vi "ZCAN_Transmit.vi"(0 "can_index_handle":u32, 1 "协议":u32(ring) items=["CAN", "CANFD"], 3 "ZCAN_Transmit_Data":T2, 5 "error in (no error)":errorcluster caption="错误输入（无错误）", 9 "ZCAN_TransmitFD_Data":T1) -> (19 "error out":errorcluster caption="错误输出")   [LabVIEW 2018]
doc: "该函数用于发送CAN报文。"
uses:
  data_type/ZCAN_Transmit_Data.ctl
  data_type/ZCAN_TransmitFD_Data.ctl
panel:
  in  "每次发送帧数（默认1）":u32=1
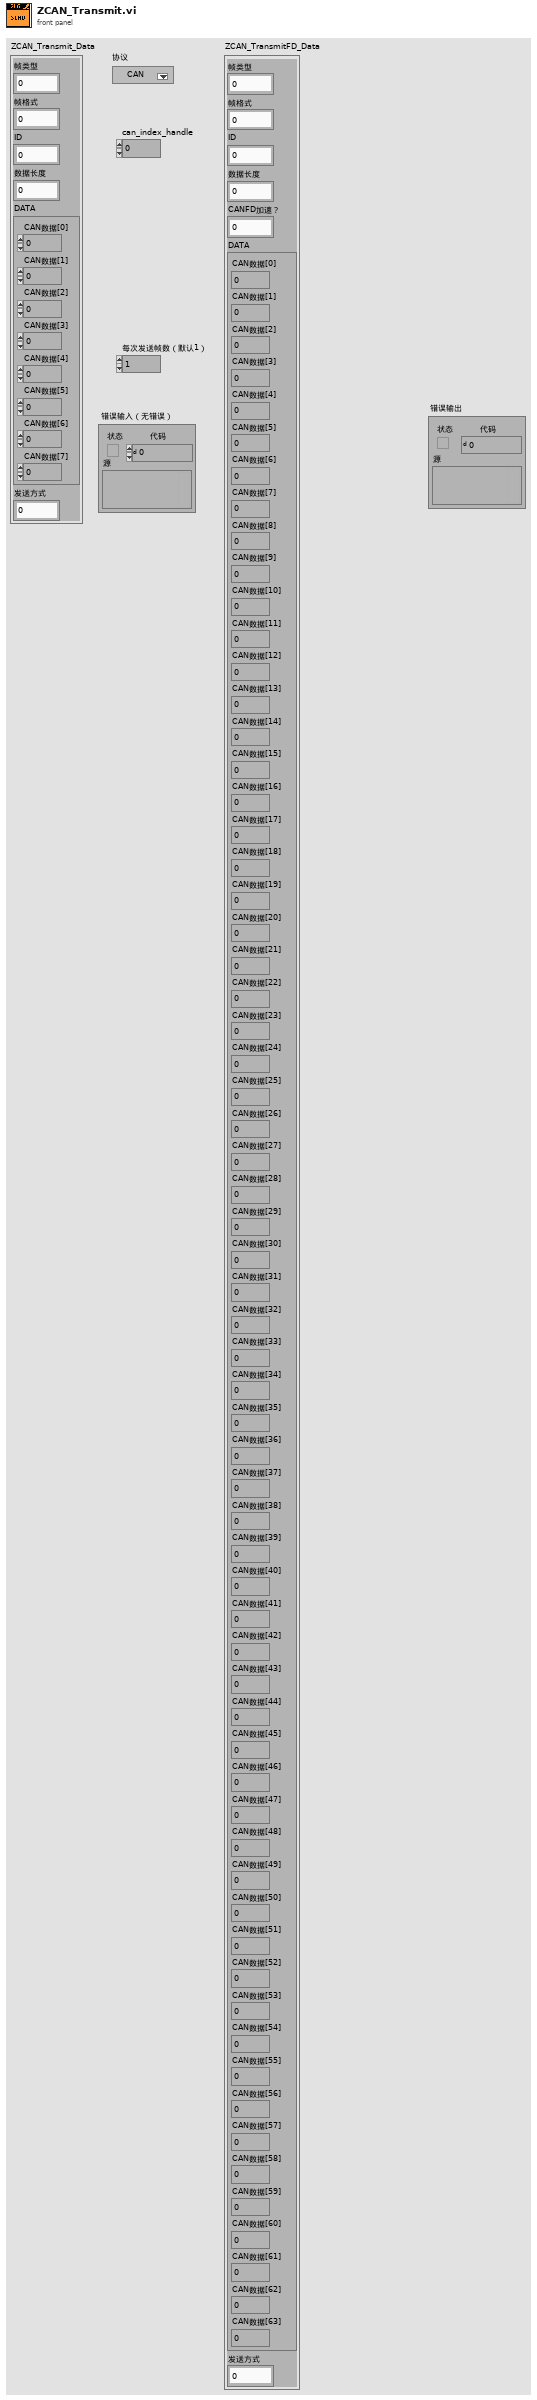
[diagram p1: front panel]
types:
  T1 = typedef "ZCAN_TransmitFD_Data.ctl" = cluster{"帧类型":u32, "帧格式":u32, "ID":u32, "数据长度":u8, "CANFD加速？":u8, "DATA":cluster{"CAN数据[0]":u8, "CAN数据[1]":u8, "CAN数据[2]":u8, "CAN数据[3]":u8, "CAN数据[4]":u8, "CAN数据[5]":u8, "CAN数据[6]":u8, "CAN数据[7]":u8, "CAN数据[8]":u8, "CAN数据[9]":u8, "CAN数据[10]":u8, "CAN数据[11] ":u8, "CAN数据[12] ":u8, "CAN数据[13] ":u8, "CAN数据[14] ":u8, "CAN数据[15] ":u8, "CAN数据[16]":u8, "CAN数据[17]":u8, "CAN数据[18]":u8, "CAN数据[19]":u8, "CAN数据[20]":u8, "CAN数据[21]":u8, "CAN数据[22]":u8, "CAN数据[23]":u8, "CAN数据[24] ":u8, "CAN数据[25]":u8, "CAN数据[26]":u8, "CAN数据[27]":u8, "CAN数据[28]":u8, "CAN数据[29]":u8, "CAN数据[30]":u8, "CAN数据[31]":u8, "CAN数据[32]":u8, "CAN数据[33]":u8, "CAN数据[34]":u8, "CAN数据[35]":u8, "CAN数据[36]":u8, "CAN数据[37]":u8, "CAN数据[38]":u8, "CAN数据[39]":u8, "CAN数据[40]":u8, "CAN数据[41]":u8, "CAN数据[42]":u8, "CAN数据[43]":u8, "CAN数据[44]":u8, "CAN数据[45]":u8, "CAN数据[46]":u8, "CAN数据[47]":u8, "CAN数据[48]":u8, "CAN数据[49]":u8, "CAN数据[50]":u8, "CAN数据[51]":u8, "CAN数据[52]":u8, "CAN数据[53]":u8, "CAN数据[54]":u8, "CAN数据[55]":u8, "CAN数据[56]":u8, "CAN数据[57]":u8, "CAN数据[58]":u8, "CAN数据[59]":u8, "CAN数据[60]":u8, "CAN数据[61]":u8, "CAN数据[62]":u8, "CAN数据[63]":u8}, "发送方式":u32}
  T2 = typedef "ZCAN_Transmit_Data.ctl" = cluster{"帧类型":u32, "帧格式":u32, "ID":u32, "数据长度":u8, "DATA":cluster{"CAN数据[0]":u8, "CAN数据[1]":u8, "CAN数据[2]":u8, "CAN数据[3]":u8, "CAN数据[4]":u8, "CAN数据[5]":u8, "CAN数据[6]":u8, "CAN数据[7]":u8}, "发送方式":u32}
  T3 = cluster{"CAN数据[0]":u8, "CAN数据[1]":u8, "CAN数据[2]":u8, "CAN数据[3]":u8, "CAN数据[4]":u8, "CAN数据[5]":u8, "CAN数据[6]":u8, "CAN数据[7]":u8, "CAN数据[8]":u8, "CAN数据[9]":u8, "CAN数据[10]":u8, "CAN数据[11] ":u8, "CAN数据[12] ":u8, "CAN数据[13] ":u8, "CAN数据[14] ":u8, "CAN数据[15] ":u8, "CAN数据[16]":u8, "CAN数据[17]":u8, "CAN数据[18]":u8, "CAN数据[19]":u8, "CAN数据[20]":u8, "CAN数据[21]":u8, "CAN数据[22]":u8, "CAN数据[23]":u8, "CAN数据[24] ":u8, "CAN数据[25]":u8, "CAN数据[26]":u8, "CAN数据[27]":u8, "CAN数据[28]":u8, "CAN数据[29]":u8, "CAN数据[30]":u8, "CAN数据[31]":u8, "CAN数据[32]":u8, "CAN数据[33]":u8, "CAN数据[34]":u8, "CAN数据[35]":u8, "CAN数据[36]":u8, "CAN数据[37]":u8, "CAN数据[38]":u8, "CAN数据[39]":u8, "CAN数据[40]":u8, "CAN数据[41]":u8, "CAN数据[42]":u8, "CAN数据[43]":u8, "CAN数据[44]":u8, "CAN数据[45]":u8, "CAN数据[46]":u8, "CAN数据[47]":u8, "CAN数据[48]":u8, "CAN数据[49]":u8, "CAN数据[50]":u8, "CAN数据[51]":u8, "CAN数据[52]":u8, "CAN数据[53]":u8, "CAN数据[54]":u8, "CAN数据[55]":u8, "CAN数据[56]":u8, "CAN数据[57]":u8, "CAN数据[58]":u8, "CAN数据[59]":u8, "CAN数据[60]":u8, "CAN数据[61]":u8, "CAN数据[62]":u8, "CAN数据[63]":u8}
  T4 = cluster{u32, "数据长度":u8, "CANFD加速？":u8, u8, u8, "DATA":cluster{"CAN数据[0]":u8, "CAN数据[1]":u8, "CAN数据[2]":u8, "CAN数据[3]":u8, "CAN数据[4]":u8, "CAN数据[5]":u8, "CAN数据[6]":u8, "CAN数据[7]":u8, "CAN数据[8]":u8, "CAN数据[9]":u8, "CAN数据[10]":u8, "CAN数据[11] ":u8, "CAN数据[12] ":u8, "CAN数据[13] ":u8, "CAN数据[14] ":u8, "CAN数据[15] ":u8, "CAN数据[16]":u8, "CAN数据[17]":u8, "CAN数据[18]":u8, "CAN数据[19]":u8, "CAN数据[20]":u8, "CAN数据[21]":u8, "CAN数据[22]":u8, "CAN数据[23]":u8, "CAN数据[24] ":u8, "CAN数据[25]":u8, "CAN数据[26]":u8, "CAN数据[27]":u8, "CAN数据[28]":u8, "CAN数据[29]":u8, "CAN数据[30]":u8, "CAN数据[31]":u8, "CAN数据[32]":u8, "CAN数据[33]":u8, "CAN数据[34]":u8, "CAN数据[35]":u8, "CAN数据[36]":u8, "CAN数据[37]":u8, "CAN数据[38]":u8, "CAN数据[39]":u8, "CAN数据[40]":u8, "CAN数据[41]":u8, "CAN数据[42]":u8, "CAN数据[43]":u8, "CAN数据[44]":u8, "CAN数据[45]":u8, "CAN数据[46]":u8, "CAN数据[47]":u8, "CAN数据[48]":u8, "CAN数据[49]":u8, "CAN数据[50]":u8, "CAN数据[51]":u8, "CAN数据[52]":u8, "CAN数据[53]":u8, "CAN数据[54]":u8, "CAN数据[55]":u8, "CAN数据[56]":u8, "CAN数据[57]":u8, "CAN数据[58]":u8, "CAN数据[59]":u8, "CAN数据[60]":u8, "CAN数据[61]":u8, "CAN数据[62]":u8, "CAN数据[63]":u8}, "发送方式":u32}
  T5 = cluster{u32, "数据长度":u8, "CANFD加速？":u8, u8, u8, "DATA":cluster{"CAN数据[0]":u8, "CAN数据[1]":u8, "CAN数据[2]":u8, "CAN数据[3]":u8, "CAN数据[4]":u8, "CAN数据[5]":u8, "CAN数据[6]":u8, "CAN数据[7]":u8, "CAN数据[8]":u8, "CAN数据[9]":u8, "CAN数据[10]":u8, "CAN数据[11] ":u8, "CAN数据[12] ":u8, "CAN数据[13] ":u8, "CAN数据[14] ":u8, "CAN数据[15] ":u8, "CAN数据[16]":u8, "CAN数据[17]":u8, "CAN数据[18]":u8, "CAN数据[19]":u8, "CAN数据[20]":u8, "CAN数据[21]":u8, "CAN数据[22]":u8, "CAN数据[23]":u8, "CAN数据[24] ":u8, "CAN数据[25]":u8, "CAN数据[26]":u8, "CAN数据[27]":u8, "CAN数据[28]":u8, "CAN数据[29]":u8, "CAN数据[30]":u8, "CAN数据[31]":u8, "CAN数据[32]":u8, "CAN数据[33]":u8, "CAN数据[34]":u8, "CAN数据[35]":u8, "CAN数据[36]":u8, "CAN数据[37]":u8, "CAN数据[38]":u8, "CAN数据[39]":u8, "CAN数据[40]":u8, "CAN数据[41]":u8, "CAN数据[42]":u8, "CAN数据[43]":u8, "CAN数据[44]":u8, "CAN数据[45]":u8, "CAN数据[46]":u8, "CAN数据[47]":u8, "CAN数据[48]":u8, "CAN数据[49]":u8, "CAN数据[50]":u8, "CAN数据[51]":u8, "CAN数据[52]":u8, "CAN数据[53]":u8, "CAN数据[54]":u8, "CAN数据[55]":u8, "CAN数据[56]":u8, "CAN数据[57]":u8, "CAN数据[58]":u8, "CAN数据[59]":u8, "CAN数据[60]":u8, "CAN数据[61]":u8, "CAN数据[62]":u8, "CAN数据[63]":u8}, "发送方式":u32}[]
  T6 = cluster{"CAN数据[0]":u8, "CAN数据[1]":u8, "CAN数据[2]":u8, "CAN数据[3]":u8, "CAN数据[4]":u8, "CAN数据[5]":u8, "CAN数据[6]":u8, "CAN数据[7]":u8}
  T7 = cluster{u32, "数据长度":u8, u8, u8, u8, "DATA":cluster{"CAN数据[0]":u8, "CAN数据[1]":u8, "CAN数据[2]":u8, "CAN数据[3]":u8, "CAN数据[4]":u8, "CAN数据[5]":u8, "CAN数据[6]":u8, "CAN数据[7]":u8}, "发送方式":u32}
  T8 = cluster{u32, "数据长度":u8, u8, u8, u8, "DATA":cluster{"CAN数据[0]":u8, "CAN数据[1]":u8, "CAN数据[2]":u8, "CAN数据[3]":u8, "CAN数据[4]":u8, "CAN数据[5]":u8, "CAN数据[6]":u8, "CAN数据[7]":u8}, "发送方式":u32}[]
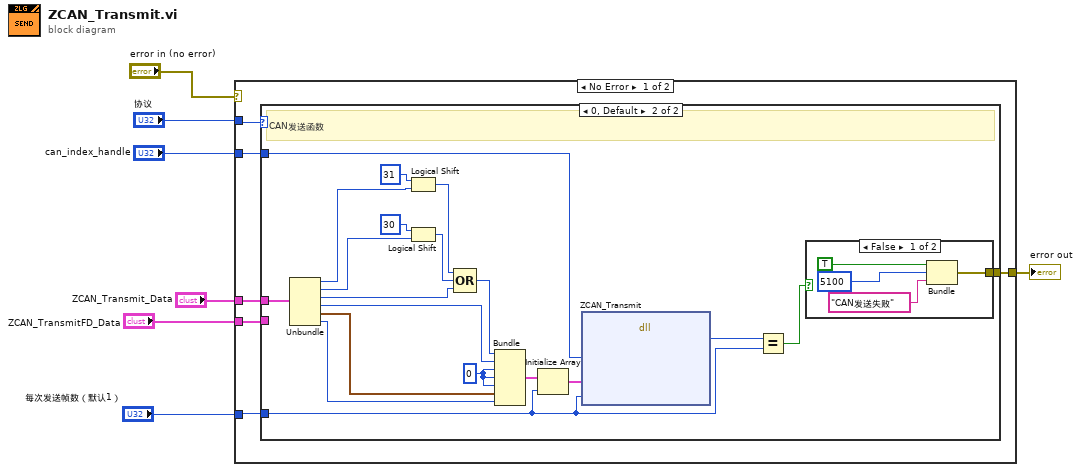
[diagram p0: block diagram]
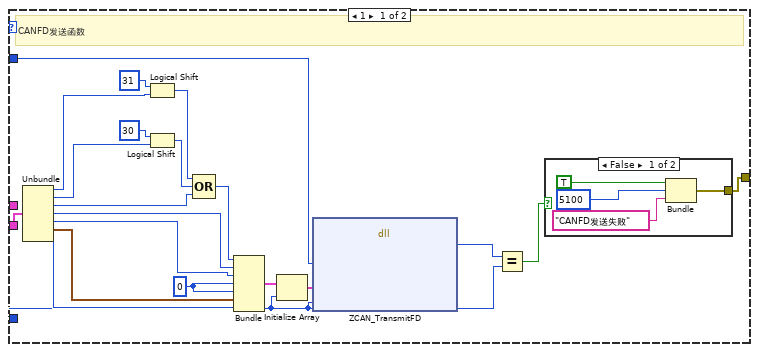
[diagram p2: hidden frame]
diagram:
  n1 = case shown="No Error" "error in (no error)" {
    selector: "error in (no error)" -> [_ w63]
    tunnel: [w13 w63] -> w6
    tunnel: "每次发送帧数（默认1）" -> [w12 _]
    tunnel: "can_index_handle" -> [w11 _]
    tunnel: "协议" -> [w10 _]
    tunnel: "ZCAN_Transmit_Data" -> [w9 _]
    tunnel: "ZCAN_TransmitFD_Data" -> [w8 _]
    frame No Error {
      n2 = case shown="0, Default" w10 {
        tunnel: [w14 w50] -> w13
        tunnel: w12 -> [w15 w49]
        tunnel: w11 -> [w20 w46]
        tunnel: w9 -> [_ w45]
        tunnel: w8 -> [w19 _]
        frame 1 {
          w34 = u8 0
          # "CANFD发送函数"
          n3 = Unbundle(w19) -> ("帧类型"=w24:u32, "帧格式"=w23:u32, "ID"=w22:u32, "数据长度"=w21:u8, "CANFD加速？"=w18:u8, "DATA"=w17:T3, "发送方式"=w16:u32)
          n4 = Logical Shift(y=i16 31, x=w24) -> (x << y=w31:u32)
          n5 = Logical Shift(y=i16 30, x=w23) -> (x << y=w28:u32)
          n6 = Compound Arithmetic op=OR ("复合运算")(w31, w28, w22) -> (w27:u32)
          n7 = Bundle ("捆绑")(w27, "数据长度"=w21, "CANFD加速？"=w18, w34, w34, "DATA"=w17, "发送方式"=w16) -> (w33:T4)  [unwired: 1 in]
          n8 = Initialize Array(w33, w15) -> (w32:T5)
          n9 = dll-call lib="PTH2\\abs CUsersadminDesktop以太网系列zlgcan_demo_CANET_TCPbinzlgcan_wrap.dll" fn="ZCAN_TransmitFD"("通道句柄"=w20, "数据帧数组"=w32, "数据帧数"=w15) -> ("返回类型"=w26:u32)  [unwired: 6 in, 2 out]
          n10 = Equal?(x=w26, y=w15) -> (x = y?=w25:bool)
          n11 = case shown="False" w25 {
            tunnel: [w35 _] -> w14
            frame False {
              n12 = Bundle("status"=TRUE, "code"=5100, "消息"="CANFD发送失败") -> (w35:cluster{"status":bool, "code":i32, "消息":string})  [unwired: 1 in]
            }
            frame True {
            }
          }
        }
        frame 0, Default {
          w58 = u8 0
          # "CAN发送函数"
          n13 = Unbundle(w45) -> ("帧类型"=w44:u32, "帧格式"=w43:u32, "ID"=w42:u32, "数据长度"=w41:u8, "DATA"=w40:T6, "发送方式"=w39:u32)
          n14 = Logical Shift(y=i16 31, x=w44) -> (x << y=w55:u32)
          n15 = Logical Shift(y=i16 30, x=w43) -> (x << y=w52:u32)
          n16 = Compound Arithmetic op=OR ("复合运算")(w55, w52, w42) -> (w51:u32)
          n17 = Bundle ("捆绑")(w51, "数据长度"=w41, w58, w58, w58, "DATA"=w40, "发送方式"=w39) -> (w57:T7)  [unwired: 1 in]
          n18 = Initialize Array(w57, w49) -> (w56:T8)
          n19 = dll-call lib="PTH2\\abs CUsersadminDesktop以太网系列zlgcan_demo_CANET_TCPbinzlgcan_wrap.dll" fn="ZCAN_Transmit"("通道句柄"=w46, "数据帧数组"=w56, "数据帧数"=w49) -> ("返回类型"=w48:u32)  [unwired: 6 in, 2 out]
          n20 = Equal?(x=w48, y=w49) -> (x = y?=w47:bool)
          n21 = case shown="False" w47 {
            tunnel: [w59 _] -> w50
            frame False {
              n22 = Bundle("status"=TRUE, "code"=5100, "消息"="CAN发送失败") -> (w59:cluster{"status":bool, "code":i32, "消息":string})  [unwired: 1 in]
            }
            frame True {
            }
          }
        }
      }
    }
    frame Error {
    }
  }
  "error out" <- w6
